vi "二进制文件（写二进制文件函数）.vi"() -> ()   [LabVIEW 2017]
panel:
  out "大小（字节）":i64
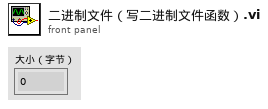
[diagram p1: front panel]
types:
  T1 = enum16{"open", "replace", "create", "open or create", "replace or create", "replace or create with confirmation"}
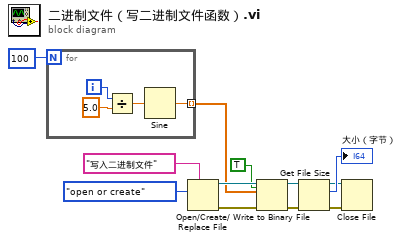
[diagram p0: block diagram]
diagram:
  n1 = for {
    N: 100 -> [_]
    tunnel: [w13] -> w7 mode=indexing
    i -> [w16]
    n2 = Divide(x=w16, y=5.0) -> (x/y=w14:dbl)
    n3 = Sine(x=w14) -> (sin(x)=w13:dbl)
  }
  n4 = Open/Create/Replace File(prompt="写入二进制文件" ("提示"), operation (0:open)=T1."open or create" ("操作(0:open)")) -> (refnum out=w9:refnum<file>, error out=w8:errorcluster)  [unwired: 4 in, 1 out]
  n5 = Write to Binary File(file (use dialog)=w9, data=w7, error in=w8, 5:TRUE ("预置数组或字符串大小？ (T)")) -> (refnum out=w5:refnum<file>, error out=w4:errorcluster)  [unwired: 2 in, 1 out]
  n6 = Get File Size(file=w5, error in=w4) -> (refnum out=w2:refnum<file>, size (in bytes)=→"大小（字节）":i64, 0:w1:errorcluster)
  n7 = Close File(refnum=w2, error in=w1) -> ()  [unwired: 2 out]
